vi "PH_TKTDS-30xx.set GUI Refs.vi"(0 "i ref in":refnum<vi>, 1 "Class":string, 2 "GUI Refs":T1, 3 "Ref PSDB Status":refnum<vi>, 5 "error in (no error)":errorcluster) -> (14 "i ref out":refnum<vi>, 19 "error out":errorcluster)   [LabVIEW 2014, in "PH_TKTDS-30xx.lvlib"]
doc: "This VI is used to set TEKTDS30xx GUI Refs; it shall be used in panels of child classes."
uses:
  PH_TKTDS-30xx.lvlib
  PH_TKTDS-30xx.GUI Refs.ctl
  PH_TKTDS-30xx.Channel Config.ctl
  PH_TKTDS-30xx.Waveform Limits.ctl
  PH_Basics/PH_PSDBWriter/PH_PSDBWriter.lvlib
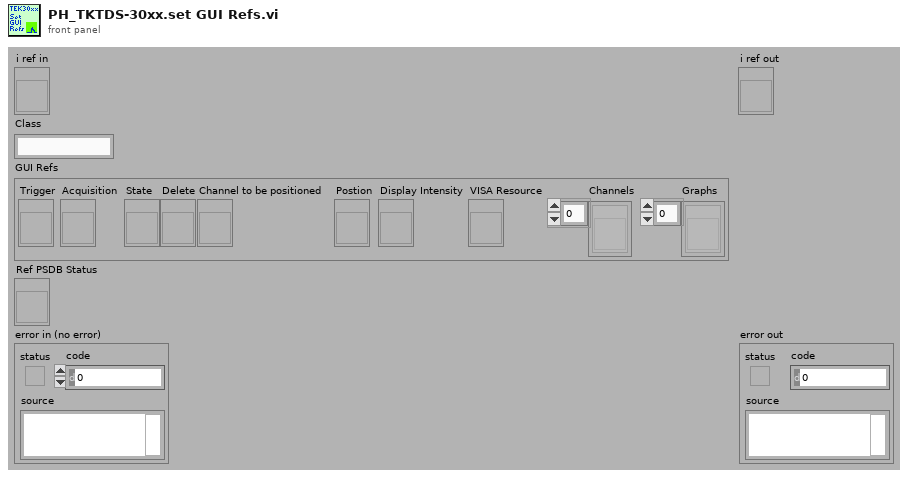
[diagram p1: front panel]
types:
  T1 = typedef "PH_TKTDS-30xx.lvlib/PH_TKTDS-30xx.GUI Refs.ctl" = cluster{"Trigger":refnum<vi>, "Acquisition":refnum<vi>, "State":refnum<vi>, "Delete":refnum<vi>, "Channel to be positioned":refnum<vi>, "Postion":refnum<vi>, "Display Intensity":refnum<vi>, "VISA Resource":refnum<vi>, "Channels":refnum<vi>[], "Graphs":refnum<vi>[]}
  T2 = typedef "PH_TKTDS-30xx.lvlib/PH_TKTDS-30xx.i attribute.ctl" = cluster{"Default VISA Resource":string, "VISA Resource Name":refnum<visa-resource-name>, "Revision":cluster{"Instrument Driver":string, "Instrument Firmware":string}, "Selftest":cluster{"Result":u32, "Message":string}, "Channels":T3[], "Trigger Configuration":T5, "Acquisition Configuration":T6, "Fetched Waveforms":T7[], "GUI Refs":T1, "State":T8, "Error Message":string, "Allow Prdc Loop?":bool}
  T3 = typedef "PH_TKTDS-30xx.lvlib/PH_TKTDS-30xx.Channel Config.ctl" = cluster{"Channel Name":string, "Input Impedance":string, "Max Input Frequency":string, "Vertical Coupling":i32, "Channel Enabled":bool, "Probe Attenuation":dbl, "Vertical Range":dbl, "Vertical Offset":dbl, "Waveform Limits":T4}
  T4 = typedef "PH_TKTDS-30xx.lvlib/PH_TKTDS-30xx.Waveform Limits.ctl" = cluster{"Start":i32, "End":i32}
  T5 = typedef "PH_TKTDS-30xx.lvlib/PH_TKTDS-30xx.Trigger Config.ctl" = cluster{"Source":string, "Slope":i32, "Level [V]":dbl}
  T6 = typedef "PH_TKTDS-30xx.lvlib/PH_TKTDS-30xx.Acquisition Config.ctl" = cluster{"Time base":dbl, "Record Length":u16, "Start Time":dbl, "Type":i32, "Continuous":bool}
  T7 = typedef "PH_TKTDS-30xx.lvlib/PH_TKTDS-30xx.fetched Waveform.ctl" = cluster{"Source":string, "Actual Points":u32, "Initial X":dbl, "X Increment":dbl, "Waveform Array":dbl[]}
  T8 = typedef "PH_StatusHandler.lvlib/PH_StatusHandler.Status.ctl" = i16
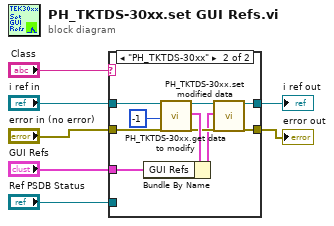
[diagram p0: block diagram]
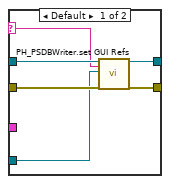
[diagram p2: hidden frame]
diagram:
  n1 = case shown="\"PH_TKTDS-30xx\"" "Class" {
    selector: "Class" -> [w9 _]
    tunnel: "error in (no error)" -> [w12 w22]
    tunnel: "i ref in" -> [w13 w21]
    tunnel: [w11 w16] -> w5
    tunnel: [w10 w15] -> w4
    tunnel: "GUI Refs" -> [_ w14]
    tunnel: "Ref PSDB Status" -> [w8 _]
    frame Default {
      n2 = call "PH_PSDBWriter.set GUI Refs.vi"("i ref in"=w13, "Class"=w9, "Ref PSDB Status"=w8, "error in"=w12) -> ("i ref out"=w11:refnum<vi>, "error out"=w10:errorcluster)  [unwired: 14 in]
    }
    frame "PH_TKTDS-30xx" {
      n3 = call "PH_TKTDS-30xx.get data to modify.vi"("i ref in"=w21, "ms timeout (10000)"=-1, "error in (no error)"=w22) -> ("i ref out"=w18:refnum<vi>, "i attribute"=w23:T2, "error out"=w19:errorcluster)  [unwired: 13 in, 1 out]
      n4 = Bundle By Name(cluster=w23, "GUI Refs"=w14) -> (w17:T2)
      n5 = call "PH_TKTDS-30xx.set modified data.vi"("i ref in"=w18, "i attribute"=w17, "error in (no error)"=w19) -> ("i ref out"=w16:refnum<vi>, "error out"=w15:errorcluster)  [unwired: 15 in]
    }
  }
  "error out" <- w4
  "i ref out" <- w5
